vi "DHE_GetCurrStatus.vi"(10 "phys. unit":string, 11 "Databse Ref":T1) -> (2 "progress":string)   [LabVIEW 2016]
uses:
  DBSHAND/private/vis/DatabaseHand_RefNum.ctl
  DBSHAND/private/vis/DatabaseHand_Element_Get(string).vi
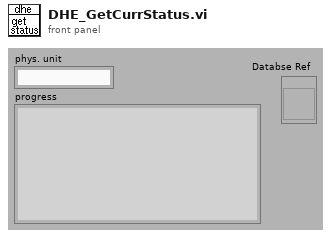
[diagram p1: front panel]
types:
  T1 = typedef "DatabaseHand_RefNum.ctl" = refnum<vi>
  T2 = enum16{"Idle", "Exposing", "Paused", "AbortExp", "Reading", "AbortRead", "FinishedReading", "Resetting", "Reducing", "Initializing"}
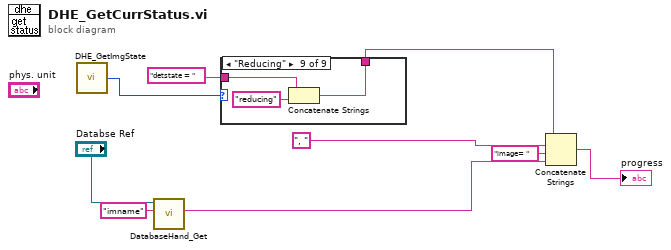
[diagram p0: block diagram]
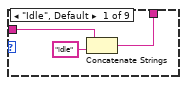
[diagram p2: hidden frame]
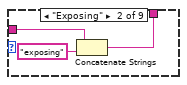
[diagram p3: hidden frame]
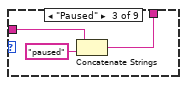
[diagram p4: hidden frame]
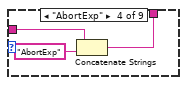
[diagram p5: hidden frame]
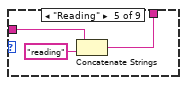
[diagram p6: hidden frame]
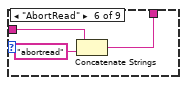
[diagram p7: hidden frame]
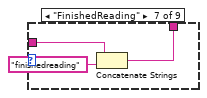
[diagram p8: hidden frame]
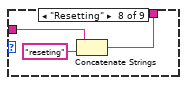
[diagram p9: hidden frame]
diagram:
  n1 = call "DHE_GetImgState.vi"() -> ("DHE_ImgState"=w1:T2)  [unwired: 9 out]
  n2 = call-poly "DatabaseHand_Get.vi"("name"="imname", "Database RefNum in"="Databse Ref") -> ("value"=w2:string)  [unwired: 3 in, 6 out]
  n3 = case shown="\"Reducing\"" w1 {
    tunnel: "detstate = " -> [w11 w15 w18 w21 w24 w27 w30 w33 w36]
    tunnel: [w10 w13 w16 w19 w22 w25 w28 w31 w34] -> w5
    frame "Idle", Default {
      n4 = Concatenate Strings(w11, "idle" ("string")) -> (w10:string)
    }
    frame "Exposing" {
      n5 = Concatenate Strings(w15, "exposing" ("string")) -> (w13:string)
    }
    frame "Paused" {
      n6 = Concatenate Strings(w18, "paused" ("string")) -> (w16:string)
    }
    frame "AbortExp" {
      n7 = Concatenate Strings(w21, "AbortExp" ("string")) -> (w19:string)
    }
    frame "Reading" {
      n8 = Concatenate Strings(w24, "reading" ("string")) -> (w22:string)
    }
    frame "AbortRead" {
      n9 = Concatenate Strings(w27, "abortread" ("string")) -> (w25:string)
    }
    frame "FinishedReading" {
      n10 = Concatenate Strings(w30, "finishedreading" ("string")) -> (w28:string)
    }
    frame "Resetting" {
      n11 = Concatenate Strings(w33, "reseting" ("string")) -> (w31:string)
    }
    frame "Reducing" {
      n12 = Concatenate Strings(w36, "reducing" ("string")) -> (w34:string)
    }
  }
  n13 = Concatenate Strings(w5, ", " ("string"), "image= " ("string"), w2) -> (→"progress":string)
